vi "WLAN_BCCEncode.vi"(8 "error in (no error)":errorcluster, 9 "BCC rate (k/n)":enum16{"1/2", "2/3", "3/4"}(ring), 10 "need add zeros?":bool, 11 "input bit stream":i8[](array[numeric])) -> (0 "error out":errorcluster, 3 "output bit stream 3":i8[](array[numeric]) caption="output bit stream")   [LabVIEW 2022 SP3]
uses:
  <vilib>/addons/Modulation/Digital/Channel Coding/MT Convolutional Encoder (Generator Matrix).vi
  <vilib>/addons/Modulation/niDMT.lvlib
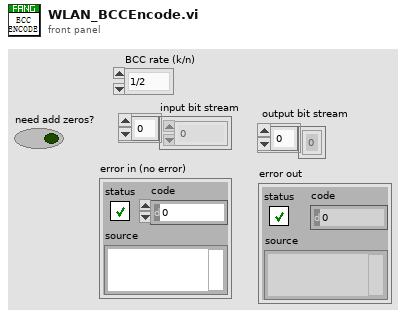
[diagram p1: front panel]
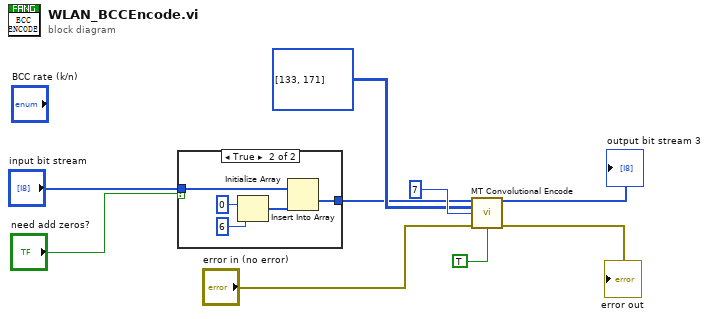
[diagram p0: block diagram]
diagram:
  n1 = case shown="True" "need add zeros?" {
    tunnel: "input bit stream" -> [w10 w12]
    tunnel: [w10 w11] -> w6
    frame False {
    }
    frame True {
      n2 = Initialize Array(i8 0 ("element"), 6 ("dimension size")) -> (w15:i8[])
      n3 = Insert Into Array(array=w12, new element=w15) -> (w11:i8[])  [unwired: 1 in]
    }
  }
  n4 = call-poly <vilib>:"MT Convolutional Encode.vi"("input bit stream"=w6, "generator matrix (n x k)"=u32[][] [[133], [171]], "constraint length (K)"=7, "error in (no error)"="error in (no error)", "reset? (T)"=TRUE) -> ("output bit stream"=→"output bit stream 3":i8[], "error out"=→"error out":errorcluster)  [unwired: 8 in, 1 out]
